vi "Arithematic_minmax_temp_convertor.vi"() -> ()   [LabVIEW 2021]
panel:
  out "Division":dbl
  out "Multiplication":dbl
  out "Substraction":dbl
  in  "stop":bool
  out "Minimum":dbl
  in  "Temp in C":dbl(slide) scale=0.0..100.0
  out "Temp in K":dbl
  out "Temp in F":dbl
  out "Maximum":dbl
  in  "C 1":dbl
  in  "B 1":dbl
  in  "A1":dbl
  out "Addition":dbl
  in  "Y":dbl
  in  "X":dbl
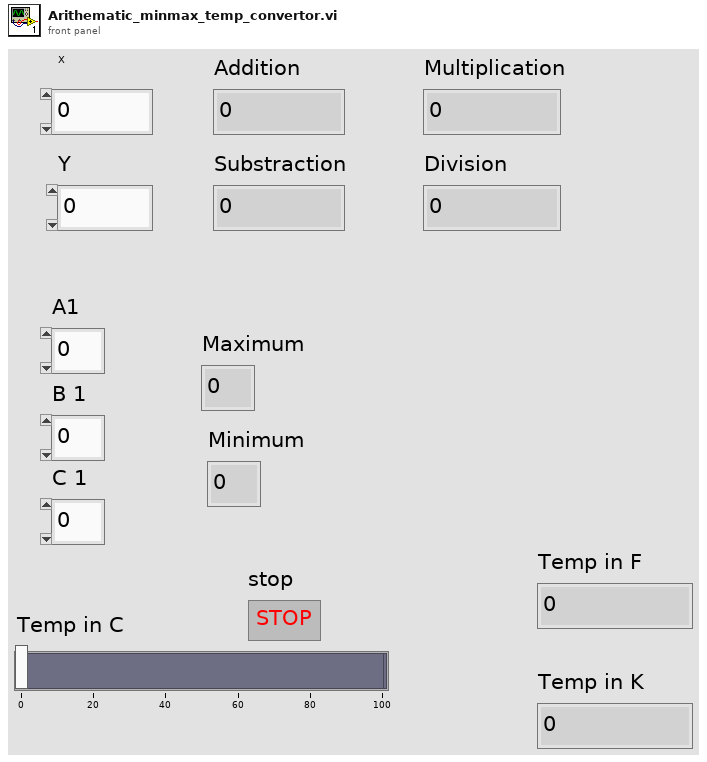
[diagram p1: front panel]
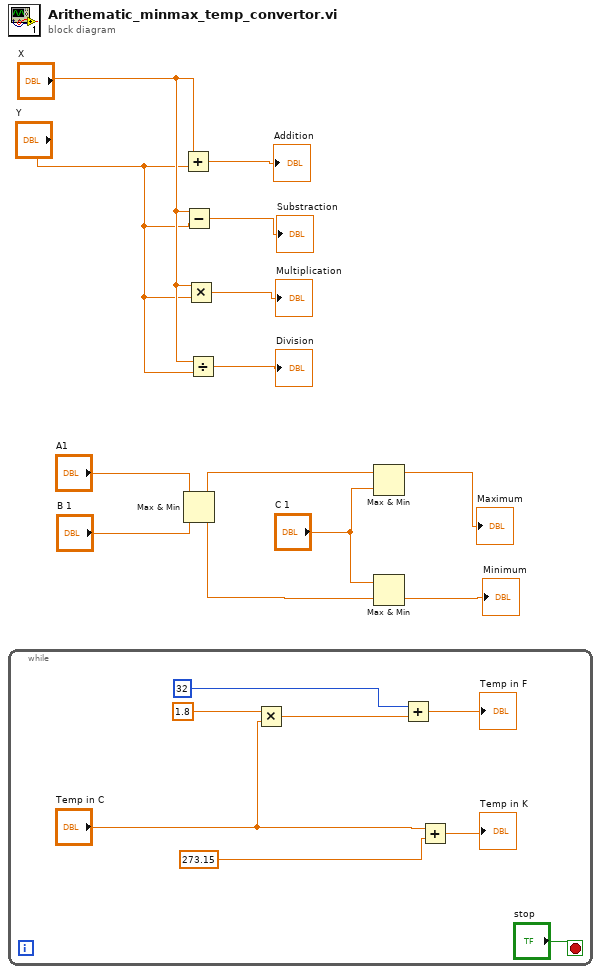
[diagram p0: block diagram]
diagram:
  n1 = while {
    stop <- "stop" stop-if-true
    n2 = Multiply(x=1.8, y="Temp in C") -> (x*y=w19:dbl)
    n3 = Add(x=32, y=w19) -> (x+y=→"Temp in F":dbl)
    n4 = Add(x="Temp in C", y=273.15) -> (x+y=→"Temp in K":dbl)
  }
  n5 = Add(x="X", y="Y") -> (x+y=→"Addition":dbl)
  n6 = Subtract(x="X", y="Y") -> (x-y=→"Substraction":dbl)
  n7 = Max & Min(x="A1", y="B 1") -> (max(x,y)=w11:dbl, min(x,y)=w9:dbl)
  n8 = Multiply(x="X", y="Y") -> (x*y=→"Multiplication":dbl)
  n9 = Divide(x="X", y="Y") -> (x/y=→"Division":dbl)
  n10 = Max & Min(x=w11, y="C 1") -> (max(x,y)=→"Maximum":dbl)  [unwired: 1 out]
  n11 = Max & Min(x="C 1", y=w9) -> (min(x,y)=→"Minimum":dbl)  [unwired: 1 out]
